vi "Files Unopen and older then hours not in use check.vi"(9 "file extention list":string[](array[string]), 10 "Dir of Files to move and FTP":path, 11 "Time (Hours) last mod must be older then":dbl) -> (3 "Files to Archive and FTP":string[][](array[string]))   [LabVIEW 2011]
doc: "Use this vi to deturmine a list of files in a directory that are have date modified dates older then the time you specify in hours, and that are currently not open by another application"
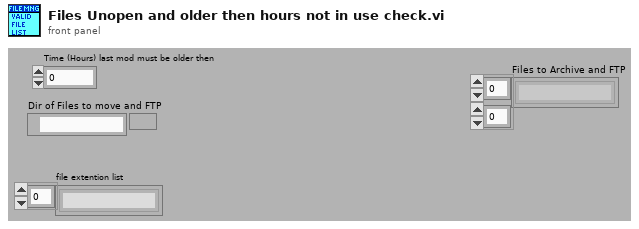
[diagram p1: front panel]
types:
  T1 = enum16{"open", "replace", "create", "open or create", "replace or create", "replace or create with confirmation"}
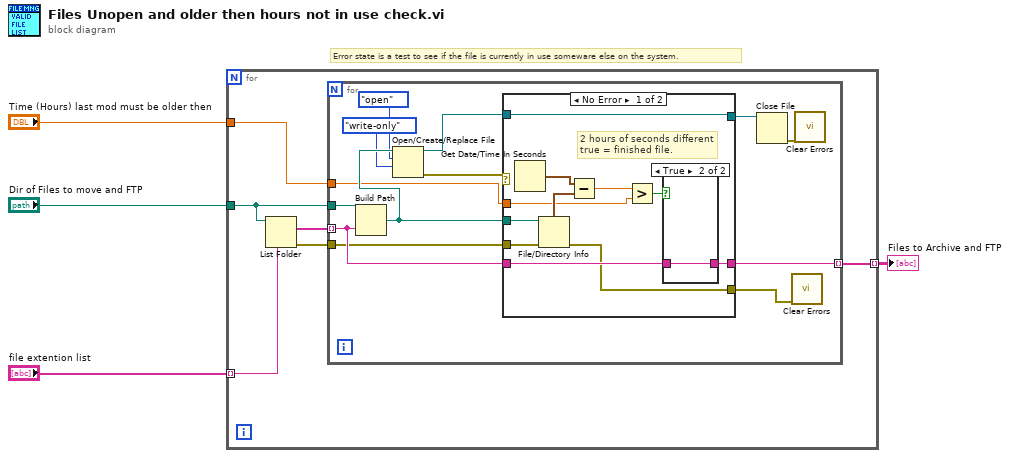
[diagram p0: block diagram]
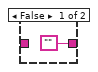
[diagram p2: hidden frame]
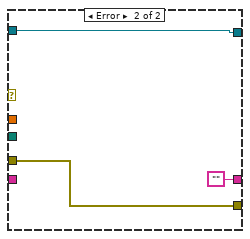
[diagram p3: hidden frame]
diagram:
  # "Error state is a test to see if the file is currently in use someware else on the system."
  n1 = for {
    tunnel: "Dir of Files to move and FTP" -> [w9]
    tunnel: "file extention list" -> [w8] mode=indexing
    tunnel: [w6] -> w1 mode=indexing
    tunnel: "Time (Hours) last mod must be older then" -> [w5]
    n2 = List Folder(path=w9, pattern=w8) -> (filenames=w10:string[], error out=w7:errorcluster)  [unwired: 2 in, 2 out]
    n3 = for {
      tunnel: w10 -> [w22] mode=indexing
      tunnel: w9 -> [w23]
      tunnel: [w21] -> w6 mode=indexing
      tunnel: w7 -> [w20]
      tunnel: w5 -> [w12]
      n4 = Build Path(base path=w23, name or relative path=w22) -> (appended path=w19:path)
      n5 = Open/Create/Replace File(file path (use dialog)=w19, operation (0:open)=T1."open", access (0:read/write)=enum16{"read/write", "read-only", "write-only"}."write-only") -> (refnum out=w15:refnum<file>, error out=w18:errorcluster)  [unwired: 3 in, 1 out]
      n6 = case shown="No Error" w18 {
        tunnel: w19 -> [w34 _]
        tunnel: w22 -> [w30 _]
        tunnel: [w29 ""] -> w21
        tunnel: w20 -> [w28 w38]
        tunnel: [w27 w38] -> w11
        tunnel: [w26 w39] -> w14
        tunnel: w15 -> [w26 w39]
        tunnel: w12 -> [w25 _]
        frame No Error {
          # "2 hours of seconds different\ntrue = finished file."
          n7 = Get Date/Time In Seconds() -> (seconds since 1Jan1904=w33:timestamp)
          n8 = File/Directory Info(path=w34, error in=w28) -> (last mod=w32:timestamp, error out=w27:errorcluster)  [unwired: 5 out]
          n9 = Subtract(x=w33, y=w32) -> (x-y=w24:dbl)
          n10 = Greater?(x=w24, y=w25) -> (0:w31:bool)
          n11 = case shown="True" w31 {
            tunnel: w30 -> [_ w36]
            tunnel: ["" w36] -> w29
            frame False {
            }
            frame True {
            }
          }
        }
        frame Error {
        }
      }
      n12 = Close File(refnum=w14) -> (error out=w13:errorcluster)  [unwired: 1 in, 1 out]
      n13 = call <vilib>:"Clear Errors.vi"("error in (no error)"=w11) -> ()  [unwired: 6 in, 1 out]
      n14 = call <vilib>:"Clear Errors.vi"("error in (no error)"=w13) -> ()  [unwired: 6 in, 1 out]
    }
  }
  "Files to Archive and FTP" <- w1
